vi "SVI_Find_nearest_in_array.vi"(2 "Search term":i32, 3 "Array":dbl[](array[numeric])) -> (0 "Difference":dbl, 1 "Index":i32)   [LabVIEW 2014]
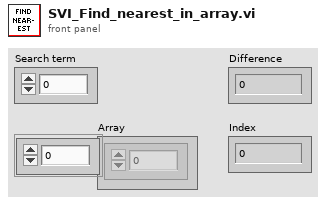
[diagram p1: front panel]
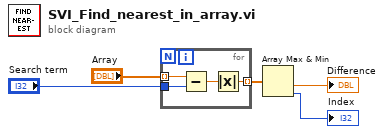
[diagram p0: block diagram]
diagram:
  n1 = for {
    tunnel: "Array" -> [w9] mode=indexing
    tunnel: "Search term" -> [w8]
    tunnel: [w6] -> w3 mode=indexing
    n2 = Subtract(x=w9, y=w8) -> (x-y=w7:dbl)
    n3 = Absolute Value(x=w7) -> (abs(x)=w6:dbl)
  }
  n4 = Array Max & Min(array=w3) -> (min value=→"Difference":dbl, min index (indices)=→"Index":i32)  [unwired: 2 out]
